vi "Compute.vi"(7 "MD5":refnum<class "MD5.lvclass">, 10 "data":u8[](array[numeric]) format="%02x") -> (2 "hash":u8[](array[numeric]) format="%02x")   [LabVIEW 2013, in "MD5.lvlib" / "MD5.lvclass"]
doc: "This VI contains the core of the MD5 algorithm."
uses:
  MD5.lvclass
  Data-vector.ctl
  K-Vector.vi
  S-Vector.vi
  F.vi
  G.vi
  H.vi
  I.vi
  T-Vector.vi
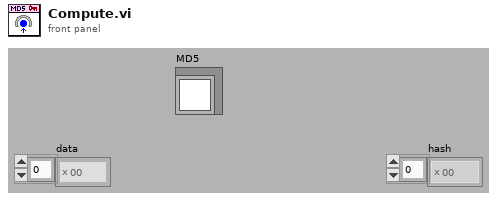
[diagram p1: front panel]
types:
  T1 = typedef "MD5.lvlib/MD5.lvclass/Data-vector.ctl" = cluster{"Data[ ]":u8[], "end":bool}
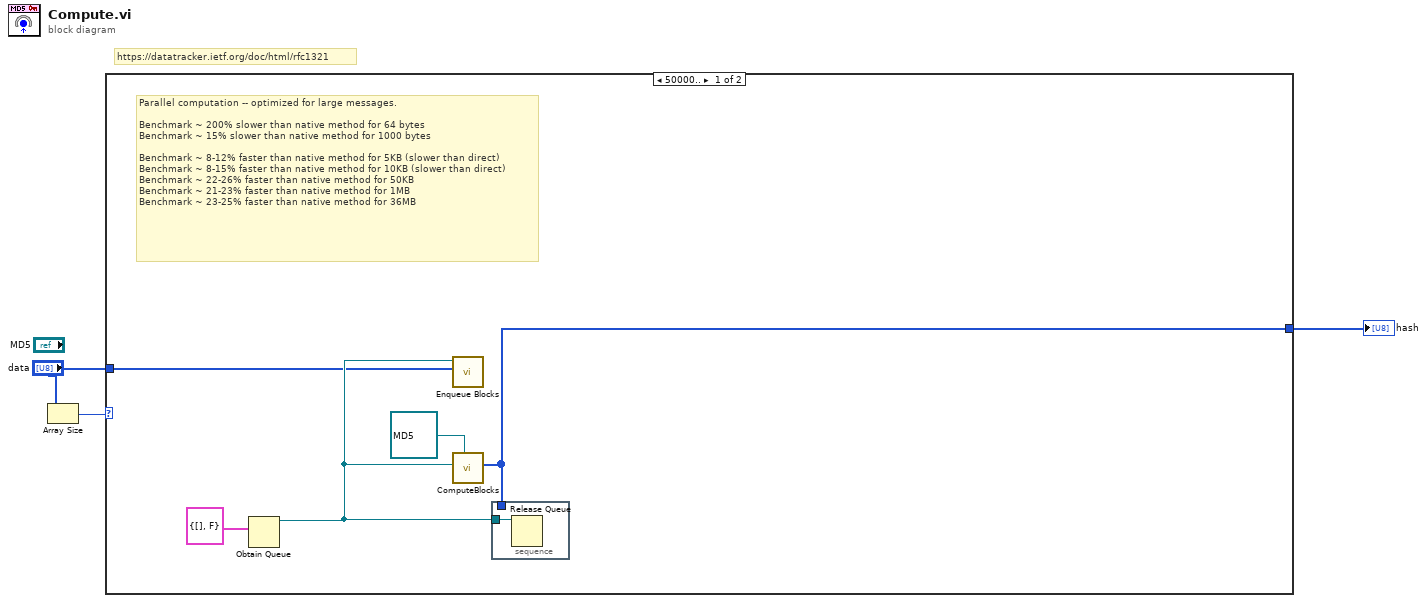
[diagram p0: block diagram]
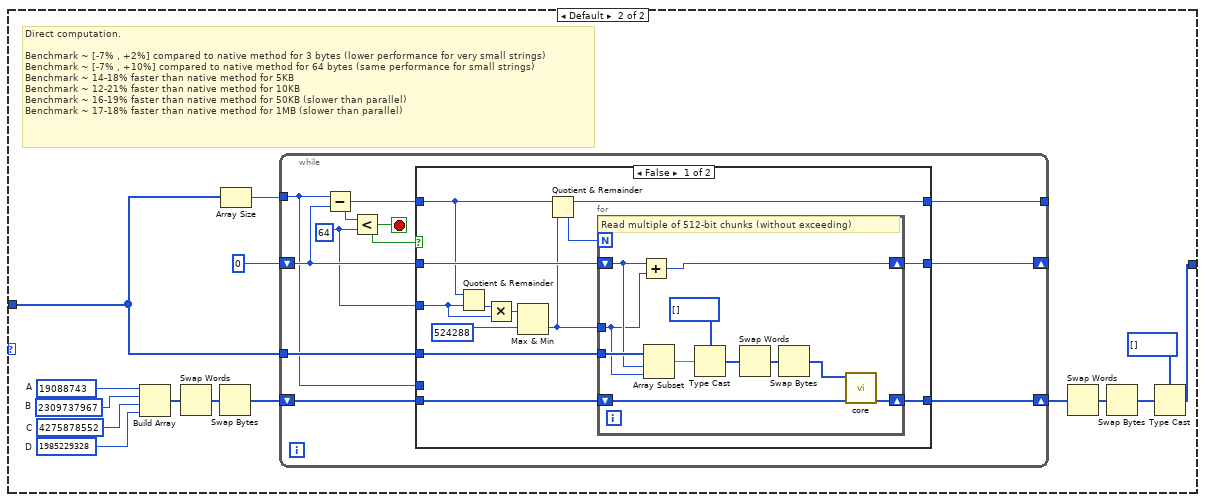
[diagram p2: hidden frame]
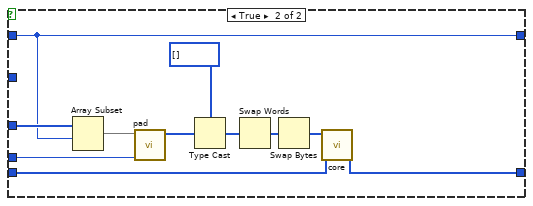
[diagram p3: hidden frame]
diagram:
  # "https://datatracker.ietf.org/doc/html/rfc1321"
  n1 = Array Size(array="data") -> (size(s)=w1:i32)
  n2 = case shown="50000.." w1 {
    tunnel: "data" -> [w5 w24]
    tunnel: [w4 w23] -> w3
    frame 50000.. {
      # "Parallel computation -- optimized for large messages.\n\nBenchmark ~ 200% slower than native method for 64 bytes\nBenchmark ~ 15% slower than native method for 1000 bytes\n\nBenchmark ~ 8-12% faster than native method for 5KB (slower than direct)\nBenchmark ~ 8-15% faster than native method for 10KB (slower than direct)\nBenchmark ~ 22-26% faster than native method for 50KB\nBenchmark ~ 21-23% faster than native method for 1MB\nBenchmark ~ 23-25% faster than native method for 36MB"
      n3 = Obtain Queue(element data type=T1 {"Data[ ]"=[], "end"=FALSE} ("cluster")) -> (queue out=w6:refnum<queue>)  [unwired: 4 in, 2 out]
      n4 = call "Enqueue Blocks.vi"("data"=w5, "Blocks queue"=w6) -> ()  [unwired: 10 in]
      n5 = call-dynamic "ComputeBlocks.vi"("MD5"=refnum<class "MD5.lvclass"> refnum ("SHA-1"), "blocks queue"=w6) -> ("hash"=w4:u8[])  [unwired: 9 in]
      n6 = stacked-sequence {
        tunnel: w6 -> [w9]
        tunnel: w4 -> [_]
        frame #0 {
          n7 = Release Queue(queue=w9) -> ()  [unwired: 2 in, 3 out]
        }
      }
    }
    frame Default {
      w17 = u32 1985229328  # D
      w18 = u32 4275878552  # C
      w19 = u32 2309737967  # B
      w20 = u32 19088743  # A
      # "Direct computation.\n\nBenchmark ~ [-7% , +2%] compared to native method for 3 bytes (lower performance for very small strings)\nBenchmark ~ [-7% , +10%] compared to native method for 64 bytes (same performance for small strings)\nBenchmark ~ 14-18% faster than native method for 5KB\nBenchmark ~ 12-21% faster than native method for 10KB\nBenchmark ~ 16-19% faster than native method for 50KB (slower than parallel)\nBenchmark ~ 17-18% faster than native method for 1MB (slower than parallel)"
      n8 = Build Array(w20, w19, w18, w17) -> (w16:u32[])
      n9 = Swap Words(1:w16) -> (0:w15:u32[])
      n10 = Swap Bytes(anything=w15) -> (byte swapped=w14:u32[])
      n11 = Array Size(array=w24) -> (size(s)=w21:i32)
      n12 = while {
        shift-right: [w30] -> _
        shift-left: 0 ("offset") -> [w32]
        tunnel: w21 -> [w25]
        tunnel: [w31] -> _
        tunnel: w24 -> [w29]
        shift-right: [w33] -> w10
        shift-left: w14 -> [w34]
        stop <- w26 stop-if-true
        w27 = 64 ("y")
        n13 = Subtract(x=w25, y=w32) -> (x-y=w28:i32)
        n14 = Less?(x=w28, y=w27) -> (x < y?=w26:bool)
        n15 = case shown="False" w26 {
          tunnel: w34 -> [w47 w60]
          tunnel: [w46 w59] -> w33
          tunnel: w32 -> [w45 w68]
          tunnel: [w39 _] -> w31
          tunnel: [w38 w68] -> w30
          tunnel: w29 -> [w37 w69]
          tunnel: w28 -> [w36 _]
          tunnel: w27 -> [w35 _]
          tunnel: w25 -> [_ w66]
          frame False {
            n16 = Quotient & Remainder(x=w36, y=w35) -> (floor(x/y)=w44:i32)  [unwired: 1 out]
            n17 = Multiply(x=w44, y=w35) -> (x*y=w43:i32)
            n18 = Max & Min(x=w43, y=524288) -> (min(x,y)=w40:i32)  [unwired: 1 out]
            n19 = Quotient & Remainder(x=w36, y=w40) -> (x-y*floor(x/y)=w39:i32, floor(x/y)=w41:i32)
            n20 = for {
              N: w41 -> [_]
              shift-right: [w50] -> w46
              shift-left: w47 -> [w51]
              shift-right: [w55] -> w38
              shift-left: w45 -> [w57]
              tunnel: w40 -> [w56]
              tunnel: w37 -> [w58]
              # "Read multiple of 512-bit chunks (without exceeding)"
              n21 = Add(x=w57, y=w56) -> (x+y=w55:i32)
              n22 = Array Subset(array=w58, index=w57, length=w56) -> (w49:u8[])
              n23 = Type Cast(type=u32[] [] ("U32"), x=w49) -> (*(type *) &x=w54:u32[])
              n24 = Swap Words(1:w54) -> (0:w48:u32[])
              n25 = Swap Bytes(anything=w48) -> (byte swapped=w52:u32[])
              n26 = call "core.vi"("ABCD in"=w51, "M[ ]"=w52) -> ("ABCD out"=w50:u32[])  [unwired: 9 in]
            }
          }
          frame True {
            n27 = Array Subset(array=w69, index=w68) -> (w67:u8[])  [unwired: 1 in]
            n28 = call "pad.vi"("data length"=w66, "Last Block"=w67) -> ("Padding"=w61:u8[])  [unwired: 8 in, 1 out]
            n29 = Type Cast(type=u32[] [] ("U32"), x=w61) -> (*(type *) &x=w62:u32[])
            n30 = Swap Words(1:w62) -> (0:w65:u32[])
            n31 = Swap Bytes(anything=w65) -> (byte swapped=w64:u32[])
            n32 = call "core.vi"("ABCD in"=w60, "M[ ]"=w64) -> ("ABCD out"=w59:u32[])  [unwired: 9 in]
          }
        }
      }
      n33 = Swap Words(1:w10) -> (0:w11:u32[])
      n34 = Swap Bytes(anything=w11) -> (byte swapped=w12:u32[])
      n35 = Type Cast(type=u8[] [], x=w12) -> (*(type *) &x=w23:u8[])
    }
  }
  "hash" <- w3
